vi "exit.vi"(8 "error in (no error)":errorcluster, 10 "Command ID":i32, 11 "CommandConstruction in":refnum<class "CommandConstruction.lvclass">) -> (0 "error out":errorcluster, 3 "CommandConstruction out":refnum<class "CommandConstruction.lvclass">)   [LabVIEW 2016, in "CommandConstruction.lvclass"]
uses:
  CommandConstruction.lvclass
  Typedefs/CommandValue.ctl
  CommandConstruction.lvclass/CommandConstruction.ctl
  ComponentTemplateCore/ComponentModel/ComponentModel/Command/Command.lvclass
  ICommandFactory/ICommandFactory.lvclass
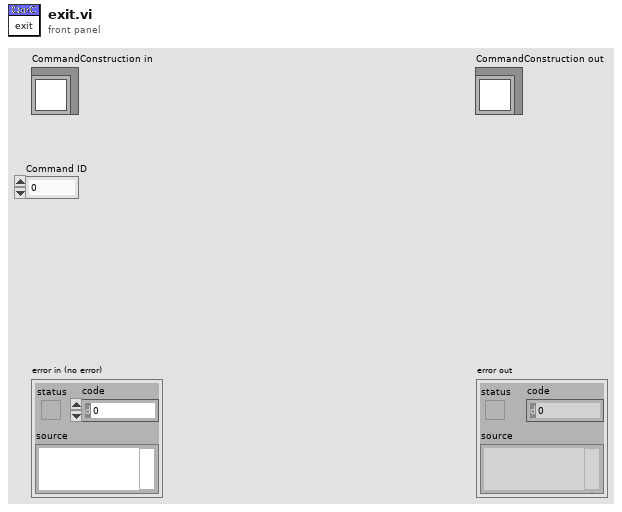
[diagram p1: front panel]
types:
  T1 = typedef "CommandValue.ctl" = enum16{"ClearError", "Disable", "Enable", "Exit", "GoToStandby", "OnHeartbeat", "OnIncomingMessagingError", "OnInterrupt", "Start"}
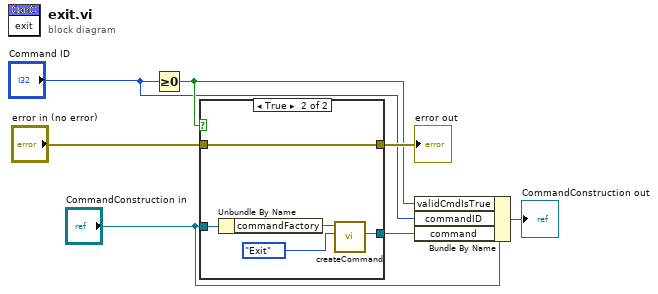
[diagram p0: block diagram]
diagram:
  n1 = Greater Or Equal To 0?(x="Command ID") -> (x >= 0?=w3:bool)
  n2 = case shown="True" w3 {
    tunnel: [w8 w10] -> w7
    tunnel: "error in (no error)" -> [w8 w10]
    tunnel: "CommandConstruction in" -> [_ w12]
    tunnel: [_ w11] -> w6
    frame False {
    }
    frame True {
      n3 = Unbundle By Name(w12) -> ("commandFactory"=w13:refnum<class "ICommandFactory.lvclass">)
      n4 = call-dynamic "createCommand.vi"("commandValue"=CommandValue."Exit", "ICommandFactory in"=w13) -> ("command"=w11:refnum<class "Command.lvclass">)  [unwired: 7 in, 2 out]
    }
  }
  "error out" <- w7
  n5 = Bundle By Name(cluster="CommandConstruction in", "validCmdIsTrue"=w3, "commandID"="Command ID", "command"=w6) -> (→"CommandConstruction out":refnum<class "CommandConstruction.lvclass">)
